vi "SignalMeas.vi"(2 "前缀":string, 3 "Data In":waveform(dbl) caption="Data_In") -> (0 "Vp-pFreq":cluster{"Vp-p":dbl, "detected frequency":dbl}, 1 "测量字符串":string)   [LabVIEW 2012]
uses:
  <vilib>/measure/matone.llb/Extract Single Tone Information 1 Chan.vi
  <vilib>/measure/mascope.llb/Cycle Average and RMS 1 chan.vi
  <vilib>/measure/mascope.llb/Amplitude and Levels 1 chan.vi
  <vilib>/measure/NI_MAPro.lvlib
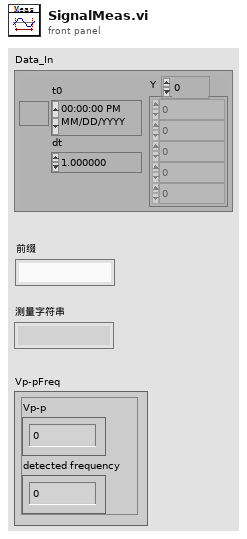
[diagram p1: front panel]
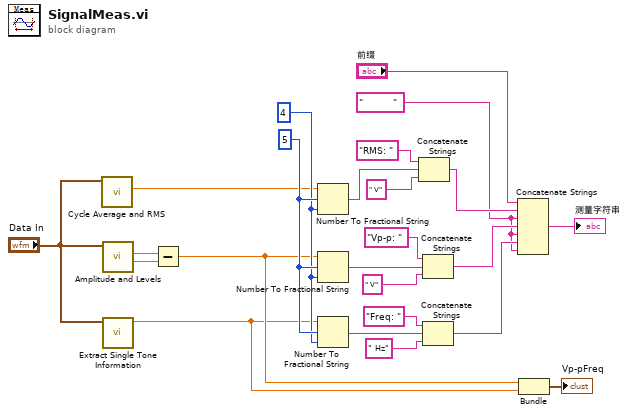
[diagram p0: block diagram]
diagram:
  w8 = 4
  w10 = "          "
  w24 = 5
  n1 = call-poly <vilib>:"Cycle Average and RMS.vi"("signal in"="Data In") -> ("cycle RMS"=w4:dbl)  [unwired: 7 in, 3 out]
  n2 = call-poly <vilib>:"Amplitude and Levels.vi"("signal in"="Data In") -> ("low state level"=w7:dbl, "high state level"=w6:dbl)  [unwired: 7 in, 2 out]
  n3 = call-poly <vilib>:"Extract Single Tone Information.vi"("time signal in"="Data In") -> ("detected frequency"=w2:dbl)  [unwired: 5 in, 5 out]
  n4 = Subtract(x=w6, y=w7) -> (x-y=w5:dbl)
  n5 = Number To Fractional String(number=w4, width (-)=w24, precision (6)=w8) -> (F-format string=w22:string)  [unwired: 1 in]
  n6 = Number To Fractional String(number=w5, width (-)=w24, precision (6)=w8) -> (F-format string=w20:string)  [unwired: 1 in]
  n7 = Number To Fractional String(number=w2, width (-)=w24, precision (6)=w8) -> (F-format string=w17:string)  [unwired: 1 in]
  n8 = Concatenate Strings("RMS: ", w22, " V") -> (w13:string)
  n9 = Concatenate Strings("Vp-p: ", w20, " V") -> (w12:string)
  n10 = Concatenate Strings("Freq: ", w17, " Hz") -> (w11:string)
  n11 = Concatenate Strings("前缀", w13, w10, w12, w10, w11, w10) -> (→"测量字符串":string)
  n12 = Bundle(w5, "detected frequency"=w2) -> (→"Vp-pFreq":cluster{dbl, "detected frequency":dbl})  [unwired: 1 in]
